vi "PushGolden.vi"(5 "isInt?":bool, 7 "Value":dbl, 8 "errin":errorcluster, 9 "SN":string, 10 "refFile":string, 11 "testnumber":enum16{"50", "40", "30", "20", "11", "10", ""}(ring)) -> (0 "error out":errorcluster)   [LabVIEW 2020]
uses:
  VarGLO/Global var.vi
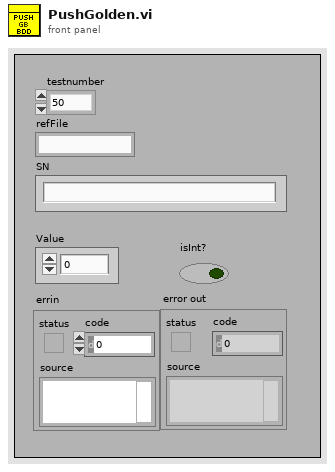
[diagram p1: front panel]
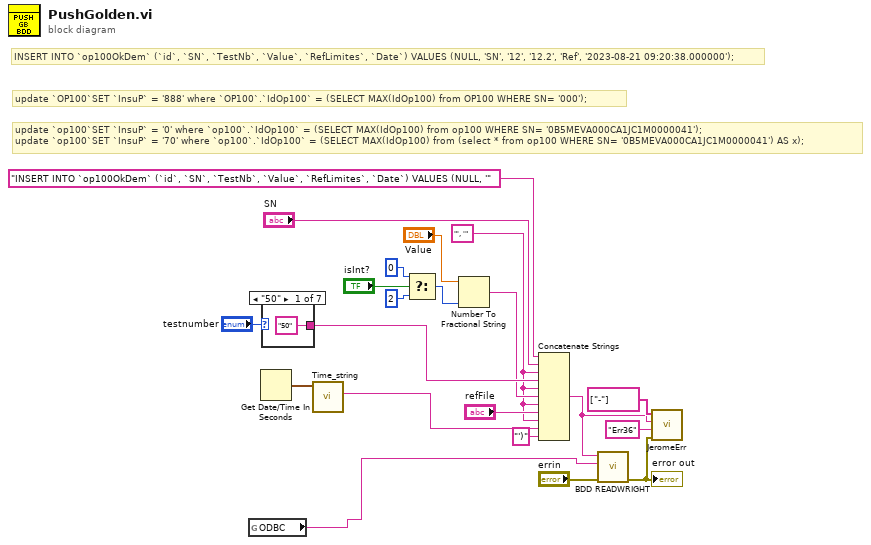
[diagram p0: block diagram]
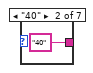
[diagram p2: hidden frame]
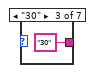
[diagram p3: hidden frame]
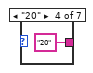
[diagram p4: hidden frame]
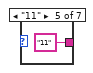
[diagram p5: hidden frame]
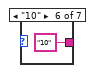
[diagram p6: hidden frame]
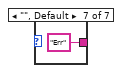
[diagram p7: hidden frame]
diagram:
  w5 = "', '" ("chaîne")
  # "INSERT INTO `op100OkDem` (`id`, `SN`, `TestNb`, `Value`, `RefLimites`, `Date`) VALUES (NULL, 'SN', '12', '12.2', 'Ref', '2023-08-21 09:20:38.000000');"
  # "update `op100`SET `InsuP` = '0' where `op100`.`IdOp100` = (SELECT MAX(IdOp100) from op100 WHERE SN= '0B5MEVA000CA1JC1M0000041');\nupdate `op100`SET `InsuP` = '70' where `op100`.`IdOp100` = (SELECT MAX(IdOp100) from (select * from op100 WHERE SN= '0B5MEVA000CA1JC1M0000041') AS x);"
  # "update `OP100`SET `InsuP` = '888' where `OP100`.`IdOp100` = (SELECT MAX(IdOp100) from OP100 WHERE SN= '000');"
  n1 = global read "Global var.vi" "ODBC"() -> (w1:string)
  n2 = Get Date/Time In Seconds() -> (seconds since 1Jan1904=w4:timestamp)
  n3 = case shown="\"50\"" "testnumber" {
    tunnel: ["50" "40" "30" "20" "11" "10" "Err"] -> w8
    frame "50" {
    }
    frame "40" {
    }
    frame "30" {
    }
    frame "20" {
    }
    frame "11" {
    }
    frame "10" {
    }
    frame "", Default {
    }
  }
  n4 = call <userlib>:"Time_string.vi"("h in"=w4) -> ("heure sql"=w3:string)  [unwired: 9 in, 1 out]
  n5 = Select ("Sélectionner")(t=i16 0 ("cas vrai"), s="isInt?", f=i16 2 ("précision (6)")) -> (s? t:f=w16:i16)
  n6 = Number To Fractional String ("Nombre en chaîne fractionnaire")(number="Value", precision (6)=w16) -> (F-format string=w7:string)  [unwired: 2 in]
  n7 = Concatenate Strings("INSERT INTO `op100OkDem` (`id`, `SN`, `TestNb`, `Value`, `RefLimites`, `Date`) VALUES (NULL, '" ("chaîne"), "SN", w5, w8, w5, w7, w5, "refFile", w5, w3, "')" ("string")) -> (w12:string)
  n8 = call <userlib>:"BDD READWRIGHT.vi"("errin"="errin", "DSN name"=w1, "Instruction"=w12) -> ("error out"=w11:errorcluster)  [unwired: 7 in, 1 out]
  "error out" <- w11
  n9 = call "JeromeErr.vi"("Errin"=w11, "CodeERR"="Err36", "RequetteSQL"=w12, "RetourSQL"=string[] ["-"]) -> ()  [unwired: 8 in]
